vi "GenerateTargetArrayFromInterval.vi"(0 "Max Range":dbl, 1 "Min Range":dbl, 2 "Left Hand":bool, 3 "Num Steps (Inclusive)":i32, 4 "Starting Position":dbl) -> (5 "Target Array":dbl[](array[numeric]))   [LabVIEW 2019]
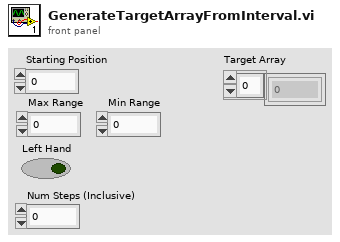
[diagram p1: front panel]
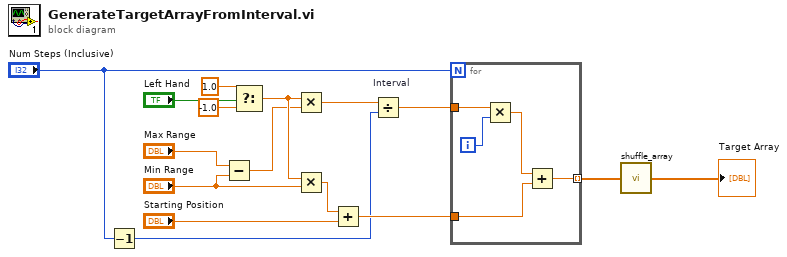
[diagram p0: block diagram]
diagram:
  n1 = Decrement(x="Num Steps (Inclusive)") -> (x-1=w1:i32)
  n2 = Subtract(x="Max Range", y="Min Range") -> (x-y=w7:dbl)
  n3 = Select(t=1.0, s="Left Hand", f=-1.0) -> (s? t:f=w8:dbl)
  n4 = Multiply(x=w8, y=w7) -> (x*y=w6:dbl)
  n5 = Multiply(x=w8, y="Min Range") -> (x*y=w5:dbl)
  n6 = Add(x=w5, y="Starting Position") -> (x+y=w3:dbl)
  n7 = Divide "Interval"(x=w6, y=w1) -> (x/y=w14:dbl)
  n8 = for {
    N: "Num Steps (Inclusive)" -> [_]
    tunnel: w14 -> [w20]
    tunnel: [w19] -> w13 mode=indexing
    tunnel: w3 -> [w17]
    i -> [w21]
    n9 = Multiply(x=w20, y=w21) -> (x*y=w18:dbl)
    n10 = Add(x=w18, y=w17) -> (x+y=w19:dbl)
  }
  n11 = call "shuffle_array.vi"("Input Array"=w13) -> ("Shuffled Array"=→"Target Array":dbl[])
